vi "Configure Gate External Source.vi"(8 "error in (no error)":errorcluster, 10 "Gate External Source (0: BNC)":i32(ring) items=["BNC", "Input 1", "Input 2"], 11 "VISA resource name":refnum<visa-resource-name>) -> (0 "error out":errorcluster, 3 "VISA resource name out":refnum<visa-resource-name>)   [LabVIEW 2024, in "Agilent 532XX Series.lvlib"]
doc: "Selects the source for external gating of measurements when advanced gating is selected. \n\n<B>Note:</B> This VI only applies to the Agilent 53220A/53230A."
uses:
  Agilent 532XX Series.lvlib
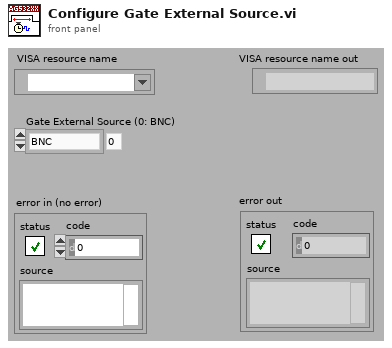
[diagram p1: front panel]
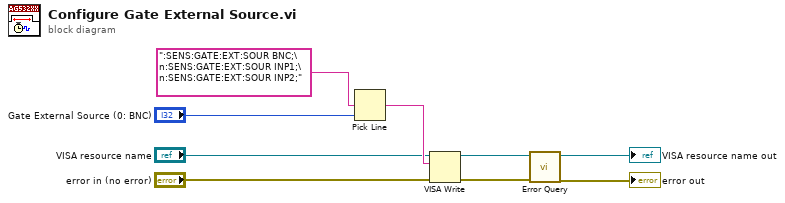
[diagram p0: block diagram]
diagram:
  n1 = Pick Line(multi-line string=":SENS:GATE:EXT:SOUR BNC;\n:SENS:GATE:EXT:SOUR INP1;\n:SENS:GATE:EXT:SOUR INP2;", line index="Gate External Source (0: BNC)") -> (output string=w7:string)  [unwired: 1 out]
  n2 = VISA Write(VISA resource name="VISA resource name", write buffer=w7, error in (no error)="error in (no error)") -> (VISA resource name out=w4:refnum<visa-resource-name>, error out=w3:errorcluster)  [unwired: 1 out]
  n3 = call "Error Query.vi"("error in (no error)"=w3, "VISA resource name"=w4) -> ("error out"=→"error out":errorcluster, "VISA resource name out"=→"VISA resource name out":refnum<visa-resource-name>)  [unwired: 8 out]
